vi "checkIffinished.vi"(9 "InDeviceState":T2, 11 "Slave tag":T1) -> (1 "OutDeviceState":T2)   [LabVIEW 2018]
uses:
  Tektronik3102/Tecktronik action loop.ctl
  tests/SlaveTag.ctl
  MasterStatus.ctl
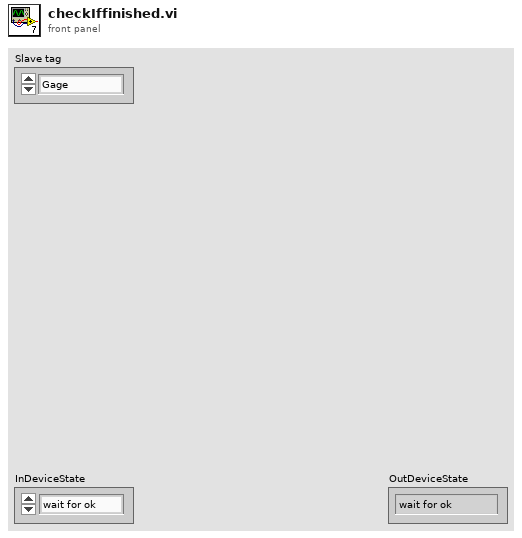
[diagram p1: front panel]
types:
  T1 = typedef "SlaveTag.ctl" = enum16{"Gage", "Tektronik", "Motors", "IC camera"}
  T2 = typedef "Tecktronik action loop.ctl" = enum16{"wait for ok", "error", "ready", "write log file", "waiting for connection", "exit", "sending command"}
  T3 = typedef "MySharedVariables.lvlib/MasterStatus.ctl" = cluster{"Camera done":bool, "Tektronik done":bool, "Motors done":bool, "Gage done":bool}[]
  T4 = cluster{"Camera done":bool, "Tektronik done":bool, "Motors done":bool, "Gage done":bool}
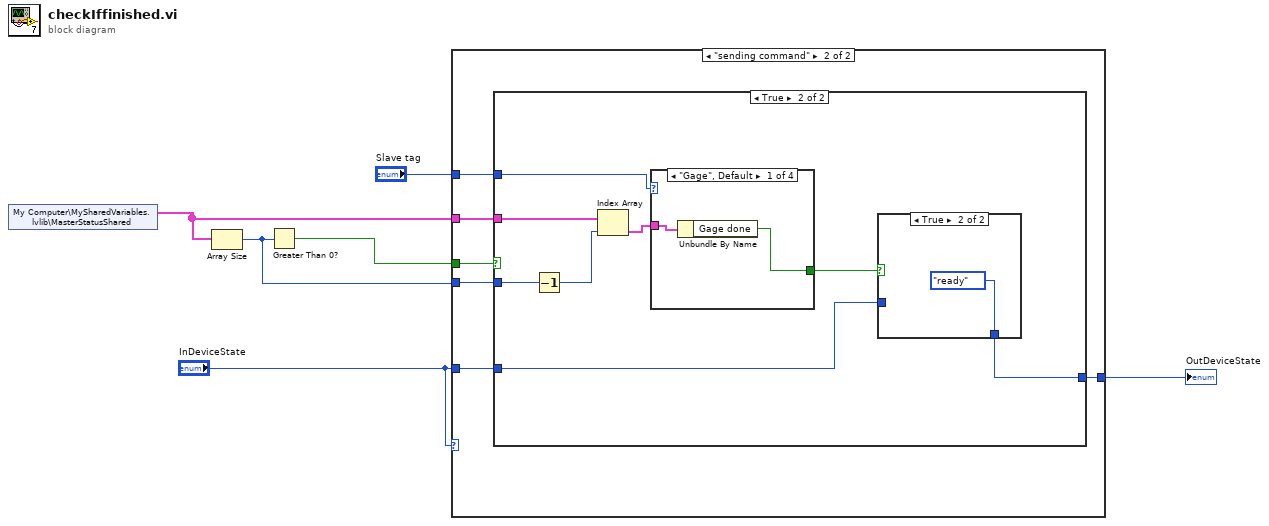
[diagram p0: block diagram]
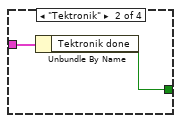
[diagram p4: hidden frame]
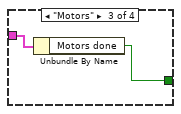
[diagram p5: hidden frame]
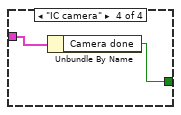
[diagram p6: hidden frame]
diagram:
  n1 = shared-variable "My Computer\\MySharedVariables.lvlib\\MasterStatusShared"() -> (w4:T3)  [unwired: 1 in, 1 out]
  n2 = Array Size(array=w4) -> (size(s)=w5:i32)
  n3 = Greater Than 0?(x=w5) -> (x > 0?=w6:bool)
  n4 = case shown="\"sending command\"" "InDeviceState" {
    tunnel: w6 -> [_ w13]
    tunnel: w5 -> [_ w12]
    tunnel: w4 -> [_ w11]
    tunnel: [w7 w10] -> w3
    tunnel: "InDeviceState" -> [w7 w9]
    tunnel: "Slave tag" -> [_ w8]
    frame Default {
    }
    frame "sending command" {
      n5 = case shown="True" w13 {
        tunnel: w12 -> [_ w18]
        tunnel: w11 -> [_ w22]
        tunnel: [w14 w20] -> w10
        tunnel: w9 -> [w14 w19]
        tunnel: w8 -> [_ w15]
        frame False {
        }
        frame True {
          n6 = Decrement(x=w18) -> (x-1=w17:i32)
          n7 = Index Array(array=w22, index=w17) -> (element=w21:T4)
          n8 = case shown="\"Gage\", Default" w15 {
            tunnel: w21 -> [w24 w26 w28 w30]
            tunnel: [w23 w25 w27 w29] -> w16
            frame "Gage", Default {
              n9 = Unbundle By Name(w24) -> ("Gage done"=w23:bool)
            }
            frame "Tektronik" {
              n10 = Unbundle By Name(w26) -> ("Tektronik done"=w25:bool)
            }
            frame "Motors" {
              n11 = Unbundle By Name(w28) -> ("Motors done"=w27:bool)
            }
            frame "IC camera" {
              n12 = Unbundle By Name(w30) -> ("Camera done"=w29:bool)
            }
          }
          n13 = case shown="True" w16 {
            tunnel: [w31 Tecktronik_action_loop."ready" ("InDeviceState")] -> w20
            tunnel: w19 -> [w31 _]
            frame False {
            }
            frame True {
            }
          }
        }
      }
    }
  }
  "OutDeviceState" <- w3
